vi "Construct.vi"(6 "Delimiter (,)":string=",", 8 "error in (no error)":errorcluster, 9 "Buffer Header Size (5000)":i32=5000, 10 "Starter Headers[]":string[](array[string]), 11 "File Path":path) -> (0 "error out":errorcluster, 3 "SLL CSV Logger out":refnum<class "SLL CSV Logger.lvclass">)   [LabVIEW 2016, in "SLL Spreadsheet.lvlib" / "SLL CSV Logger.lvclass"]
doc: "Constructs the CSV Logger Object with the logger path, delimiter and the initial header list. \n\nThe header list is optional. New headers can be dynamically added during logging as well."
uses:
  SLL CSV Logger.lvclass
  SLL CSV Logger.lvclass/SLL CSV Logger.ctl
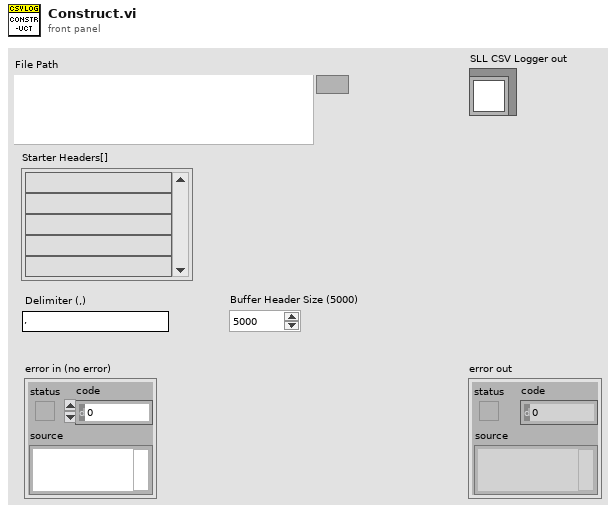
[diagram p1: front panel]
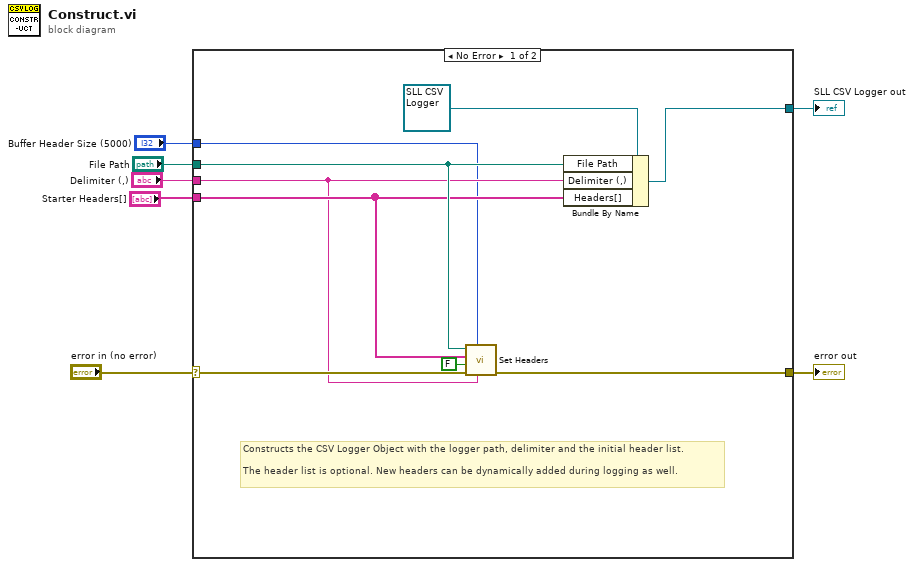
[diagram p0: block diagram]
diagram:
  n1 = case shown="No Error" "error in (no error)" {
    selector: "error in (no error)" -> [w14 w17]
    tunnel: [w13 w17] -> w6
    tunnel: [w15 _] -> w5
    tunnel: "File Path" -> [w12 _]
    tunnel: "Delimiter (,)" -> [w10 _]
    tunnel: "Starter Headers[]" -> [w11 _]
    tunnel: "Buffer Header Size (5000)" -> [w8 _]
    frame No Error {
      # "Constructs the CSV Logger Object with the logger path, delimiter and the initial header list. \n\nThe header list is optional. New headers can be dynamically added during logging as well."
      n2 = call "Set Headers.vi"("Delimiter (,)"=w10, "Buffer Header Size (5,000)"=w8, "error in (no error)"=w14, "Update Existing? (T)"=FALSE ("Update Existing? (F)"), "Headers[]"=w11, "File Path"=w12) -> ("error out"=w13:errorcluster)  [unwired: 4 in, 1 out]
      n3 = Bundle By Name(cluster=refnum<class "SLL CSV Logger.lvclass"> refnum ("SLL Spreadsheet Logger in"), "File Path"=w12, "Delimiter (,)"=w10, "Headers[]"=w11) -> (w15:refnum<class "SLL CSV Logger.lvclass">)
    }
    frame Error {
    }
  }
  "error out" <- w6
  "SLL CSV Logger out" <- w5
